vi "LV86_BuildMask.vi"(2 "ROI":T2, 3 "Image":T1 {"Dialogs" format="%.0b"}) -> (1 "Image":T1 {"Dialogs" format="%.0b"})   [LabVIEW 2024]
doc: "This vi will return a mask. The area inside the defined ROI is filled with 1 and the rest of the image is set to 0."
uses:
  <userlib>/ImageProcessing/QTLIB_2595_LV86/QT_Image.ctl
panel:
  # "This vi will return a mask.  The area inside the defined ROI is filled with 1 and the rest of the image is set to 0."
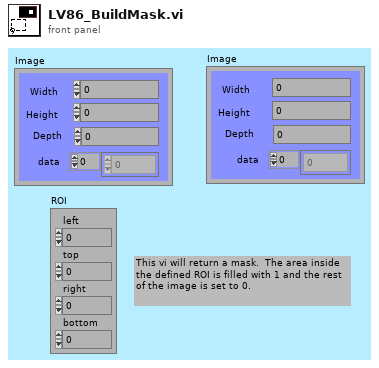
[diagram p1: front panel]
types:
  T1 = typedef "QT_Image.ctl" = cluster{"Width":i32, "Height":i32, "Depth":i32, "data":u8[], "Compressed data":u8[], "Color table":u32[], "Duration":i32, "Options":i32, "Timestamp":i32, "ID":i32, "Reserved":i32, "Dialogs":u32}
  T2 = cluster{"left":i32, "top":i32, "right":i32, "bottom":i32}
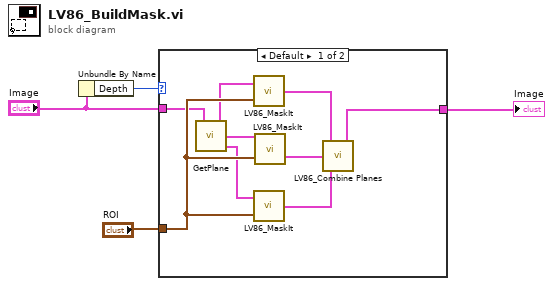
[diagram p0: block diagram]
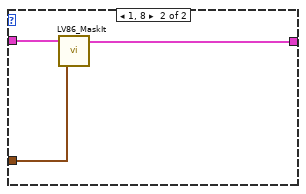
[diagram p2: hidden frame]
diagram:
  n1 = Unbundle By Name("Image") -> ("Depth"=w1:i32)
  n2 = case shown="Default" w1 {
    tunnel: "ROI" -> [w13 w16]
    tunnel: [w5 w15] -> w3
    tunnel: "Image" -> [w12 w14]
    frame Default {
      n3 = call <userlib>:"GetPlane.vi"("Image In"=w12) -> ("Blue Plane Out"=w9:T1, "Green Plane Out"=w10:T1, "Red Plane Out"=w11:T1)
      n4 = call <userlib>:"LV86_MaskIt.vi"("ROI"=w13, "Image In"=w11) -> ("Image Out"=w8:T1)
      n5 = call <userlib>:"LV86_MaskIt.vi"("ROI"=w13, "Image In"=w9) -> ("Image Out"=w6:T1)
      n6 = call <userlib>:"LV86_MaskIt.vi"("ROI"=w13, "Image In"=w10) -> ("Image Out"=w7:T1)
      n7 = call <userlib>:"LV86_Combine Planes.vi"("Blue"=w6, "Green"=w7, "Red"=w8) -> ("Image 2"=w5:T1)  [unwired: 1 out]
    }
    frame 1, 8 {
      n8 = call <userlib>:"LV86_MaskIt.vi"("ROI"=w16, "Image In"=w14) -> ("Image Out"=w15:T1)
    }
  }
  "Image" <- w3
